vi "New Child.vi"(8 "error in (no error)":errorcluster, 10 "Child Token":string, 11 "PathTreeNode in":refnum<class "PathTreeNode.lvclass">) -> (0 "error out":errorcluster, 2 "Child":refnum<class "PathTreeNode.lvclass">, 3 "PathTreeNode out":refnum<class "PathTreeNode.lvclass">)   [LabVIEW 2020, in "PathTree.lvlib" / "PathTreeNode.lvclass"]
uses:
  PathTreeNode.lvclass
  PathTreeNode.lvclass/PathTreeNode.ctl
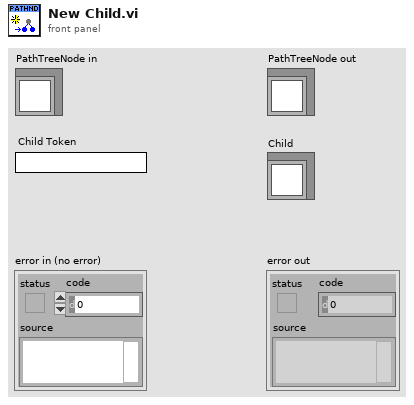
[diagram p1: front panel]
types:
  T1 = typedef "Advanced Structures.lvlib/PathTreeNode.lvclass/Ref Data.ctl" = cluster{"Tree":refnum<class>, "Parent":refnum<class>, "Token":string, "Child Tokens":string[], "Child Nodes":refnum<class>[], "Value":refnum<class>, "Has Value":bool}
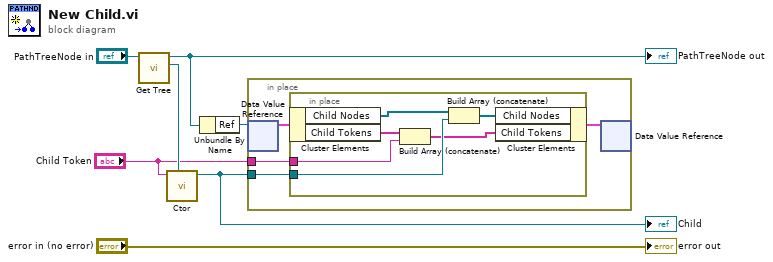
[diagram p0: block diagram]
diagram:
  n1 = call "Get Tree.vi"("PathTreeNode in"="PathTreeNode in") -> ("Tree"=w5:refnum<class "PathTree.lvclass">, "PathTreeNode out"=w1:refnum<class "PathTreeNode.lvclass">)  [unwired: 8 in, 1 out]
  "PathTreeNode out" <- w1
  n2 = call "Ctor.vi"("Tree"=w5, "Token"="Child Token") -> ("PathTreeNode out"=w3:refnum<class "PathTreeNode.lvclass">)  [unwired: 8 in, 1 out]
  "Child" <- w3
  n3 = Unbundle By Name(w1) -> ("Ref"=w4:refnum<data-value>)
  n4 = in-place {
    in-place-border: w3 -> [w9]
    in-place-border: "Child Token" -> [w8]
    n5 = in-place-dvr #1(w4) -> (w11:T1)  [unwired: 1 out]
    n6 = in-place {
      in-place-border: w9 -> [w13]
      in-place-border: w8 -> [w16]
      n7 = in-place-cluster #2(w11) -> ("Child Nodes"=w15:refnum<class>[], "Child Tokens"=w17:string[])
      n8 = Build Array (concatenate)(w17, w16) -> (w12:string[])
      n9 = Build Array (concatenate)(w15, w13) -> (w14:refnum<class>[])
      n10 = in-place-cluster #2("Child Nodes"=w14, "Child Tokens"=w12) -> (w10:T1)
    }
    n11 = in-place-dvr #1(w10) -> ()  [unwired: 2 out]
  }
  "error out" <- "error in (no error)"
